vi "MECC CRC32_2011.vi"(8 "error in (no error)":errorcluster, 10 "CRCBuffer":u32=4294967295 format="%x", 11 "FileToCalculate":path) -> (0 "error out":errorcluster, 2 "CRC32Value":u32 format="%x")   [LabVIEW 2016]
panel:
  # "CRC32 Calculator\nSelect a file for FileToCalculate and run."
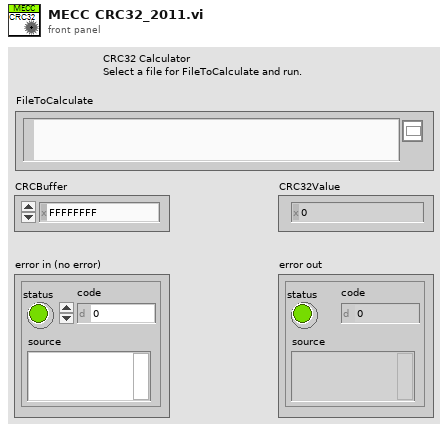
[diagram p1: front panel]
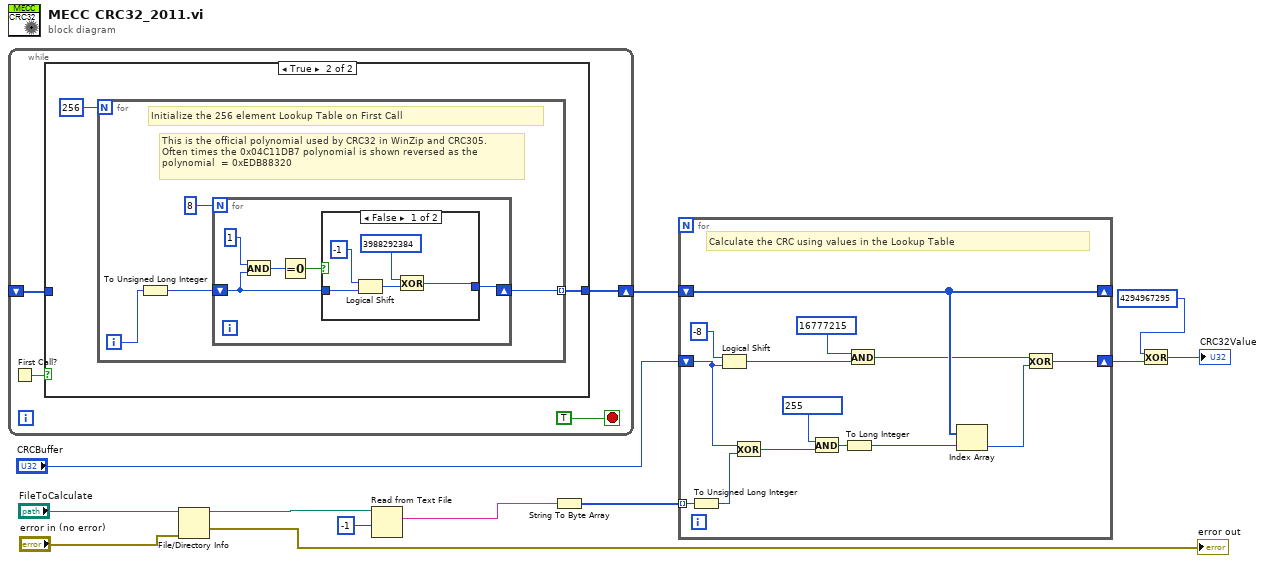
[diagram p0: block diagram]
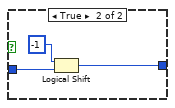
[diagram p3: hidden frame]
diagram:
  n1 = while {
    shift-right: [w15] -> w2
    shift-left: _ -> [w14]
    stop <- TRUE stop-if-true
    n2 = First Call?() -> (First Call?: T/F=w16:bool)
    n3 = case shown="True" w16 {
      tunnel: [w17 w18] -> w15
      tunnel: w14 -> [w17 _]
      frame False {
      }
      frame True {
        n4 = for {
          N: 256 -> [_]
          tunnel: [w22] -> w18 mode=indexing
          i -> [w21]
          # "Initialize the 256 element Lookup Table on First Call"
          # "This is the official polynomial used by CRC32 in WinZip and CRC305.\nOften times the 0x04C11DB7 polynomial is shown reversed as the\npolynomial  = 0xEDB88320"
          n5 = To Unsigned Long Integer(number=w21) -> (unsigned 32bit integer=w20:u32)
          n6 = for {
            N: 8 -> [_]
            shift-right: [w28] -> w22
            shift-left: w20 -> [w27]
            n7 = And(x=u32 1, y=w27) -> (x .and. y?=w26:u32)
            n8 = Equal To 0?(x=w26) -> (x = 0?=w24:bool)
            n9 = case shown="False" w24 {
              tunnel: w27 -> [w33 w36]
              tunnel: [w29 w34] -> w28
              frame False {
                n10 = Logical Shift(y=-1, x=w33) -> (x << y=w31:u32)
                n11 = Exclusive Or(1:w31, 2:u32 3988292384) -> (0:w29:u32)
              }
              frame True {
                n12 = Logical Shift(y=-1, x=w36) -> (x << y=w34:u32)
              }
            }
          }
        }
      }
    }
  }
  n13 = File/Directory Info(path="FileToCalculate", error in="error in (no error)") -> (path out=w6:path, error out=→"error out":errorcluster)  [unwired: 5 out]
  n14 = Read from Text File(file (use dialog)=w6, count=-1) -> (text=w1:string)  [unwired: 2 in, 3 out]
  n15 = String To Byte Array(string=w1) -> (unsigned byte array=w11:u8[])
  n16 = for {
    tunnel: w11 -> [w50] mode=indexing
    shift-right: [w43] -> w5
    shift-left: "CRCBuffer" -> [w39]
    shift-right: [w42] -> _
    shift-left: w2 -> [w42]
    # "Calculate the CRC using values in the Lookup Table"
    n17 = To Unsigned Long Integer(number=w50) -> (unsigned 32bit integer=w49:u32)
    n18 = Logical Shift(y=-8, x=w39) -> (x << y=w44:u32)
    n19 = Exclusive Or(1:w49, 2:w39) -> (0:w47:u32)
    n20 = And(x=u32 255, y=w47) -> (x .and. y?=w38:u32)
    n21 = To Long Integer(number=w38) -> (32bit integer=w46:i32)
    n22 = And(x=u32 16777215, y=w44) -> (x .and. y?=w41:u32)
    n23 = Index Array "Index Array"(array=w42, index=w46) -> (element=w45:u32)
    n24 = Exclusive Or(1:w45, 2:w41) -> (0:w43:u32)
  }
  n25 = Exclusive Or(1:w5, 2:u32 4294967295) -> (0:→"CRC32Value":u32)
